vi "1.-Cubo RGB.vi"() -> ()   [LabVIEW 2020]
panel:
  out "new picture 6":picture
  out "RGB Cube Bottom":picture
  out "RGB Cube Right":picture
  out "RGB Cube Front":picture
  out "RGB Cube Left":picture
  out "RGB Cube Top":picture
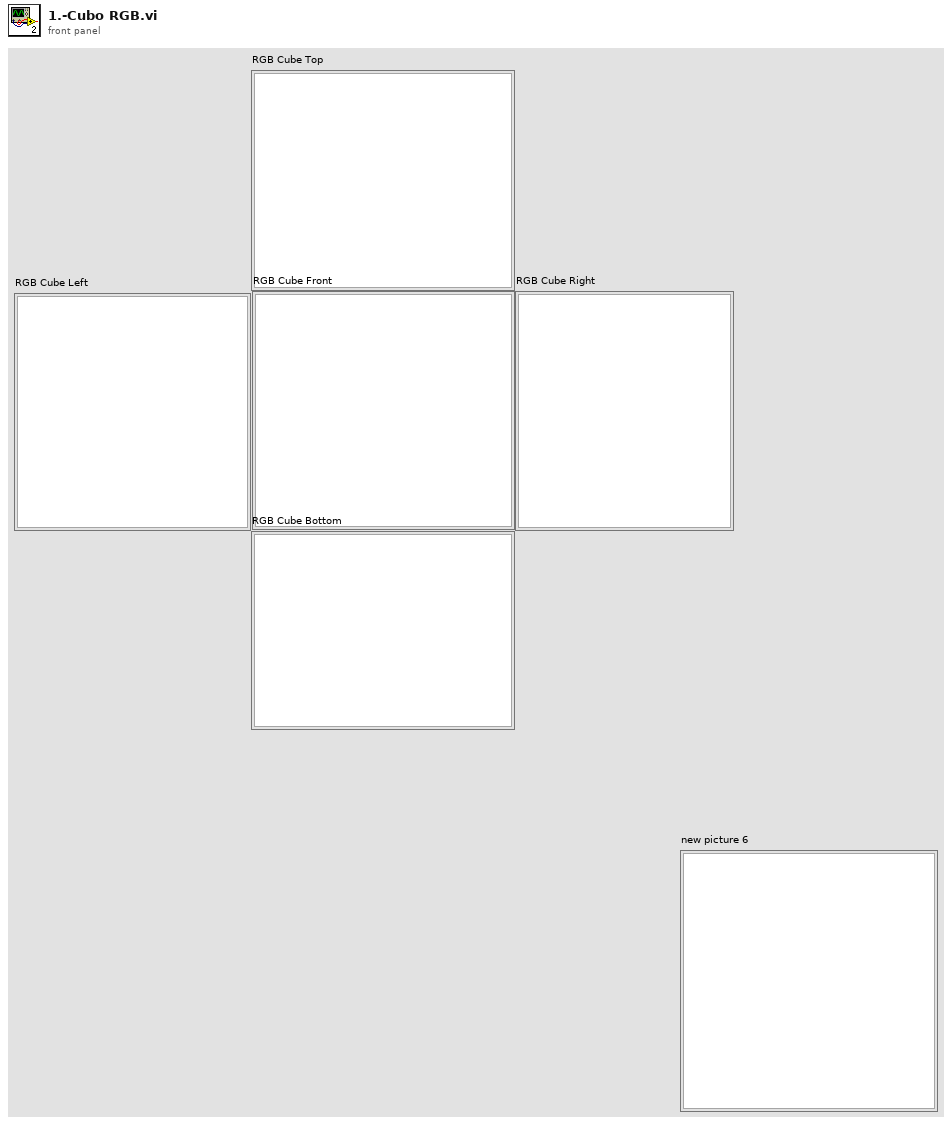
[diagram p1: front panel]
types:
  T1 = typedef "imagedata.ctl" = cluster{"image type":i32, "image depth":i32, "image":u8[], "mask":u8[], "colors":u32[], "Rectangle":cluster{"left":i16, "top":i16, "right":i16, "bottom":i16}}
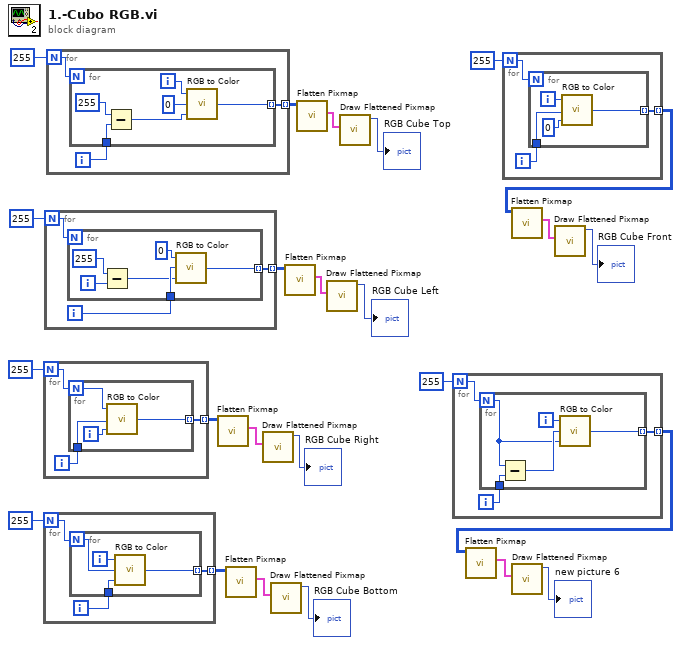
[diagram p0: block diagram]
diagram:
  n1 = for {
    N: 255 -> [w25]
    tunnel: [w26] -> w9 mode=indexing
    i -> [w27]
    n2 = for {
      N: w25 -> [w29]
      tunnel: w27 -> [w30]
      tunnel: [w31] -> w26 mode=indexing
      i -> [w28]
      n3 = call <vilib>:"RGB to Color.vi"("B"=w28, "G"=w30, "R"=w29) -> ("Color"=w31:u32)
    }
  }
  n4 = for {
    N: 255 -> [w32]
    tunnel: [w33] -> w5 mode=indexing
    i -> [w34]
    n5 = for {
      N: w32 -> [w36]
      tunnel: w34 -> [w35]
      tunnel: [w38] -> w33 mode=indexing
      i -> [w37]
      n6 = call <vilib>:"RGB to Color.vi"("B"=w35, "G"=w36, "R"=w37) -> ("Color"=w38:u32)
    }
  }
  n7 = for {
    N: 255 -> [w39]
    tunnel: [w40] -> w17 mode=indexing
    i -> [w41]
    n8 = for {
      N: w39 -> [_]
      tunnel: w41 -> [w44]
      tunnel: [w47] -> w40 mode=indexing
      i -> [w43]
      n9 = Subtract(x=255, y=w43) -> (x-y=w42:i32)
      n10 = call <vilib>:"RGB to Color.vi"("B"=w42, "G"=w44, "R"=0) -> ("Color"=w47:u32)
    }
  }
  n11 = for {
    N: 255 -> [w48]
    tunnel: [w49] -> w21 mode=indexing
    i -> [w50]
    n12 = for {
      N: w48 -> [_]
      tunnel: w50 -> [w53]
      tunnel: [w55] -> w49 mode=indexing
      i -> [w56]
      n13 = Subtract(x=255, y=w53) -> (x-y=w51:i32)
      n14 = call <vilib>:"RGB to Color.vi"("B"=w51, "G"=0, "R"=w56) -> ("Color"=w55:u32)
    }
  }
  n15 = call <vilib>:"Flatten Pixmap.vi"("24-bit pixmap"=w9) -> ("image data"=w11:T1)  [unwired: 10 in]
  n16 = call <vilib>:"Flatten Pixmap.vi"("24-bit pixmap"=w5) -> ("image data"=w7:T1)  [unwired: 10 in]
  n17 = call <vilib>:"Draw Flattened Pixmap.vi"("image data"=w11) -> ("new picture"=→"RGB Cube Right":picture)  [unwired: 8 in]
  n18 = call <vilib>:"Draw Flattened Pixmap.vi"("image data"=w7) -> ("new picture"=→"RGB Cube Bottom":picture)  [unwired: 8 in]
  n19 = call <vilib>:"Flatten Pixmap.vi"("24-bit pixmap"=w17) -> ("image data"=w19:T1)  [unwired: 10 in]
  n20 = call <vilib>:"Flatten Pixmap.vi"("24-bit pixmap"=w21) -> ("image data"=w23:T1)  [unwired: 10 in]
  n21 = call <vilib>:"Draw Flattened Pixmap.vi"("image data"=w19) -> ("new picture"=→"RGB Cube Left":picture)  [unwired: 8 in]
  n22 = call <vilib>:"Draw Flattened Pixmap.vi"("image data"=w23) -> ("new picture"=→"RGB Cube Top":picture)  [unwired: 8 in]
  n23 = for {
    N: 255 -> [w57]
    tunnel: [w58] -> w1 mode=indexing
    i -> [w59]
    n24 = for {
      N: w57 -> [w60]
      tunnel: w59 -> [w61]
      tunnel: [w64] -> w58 mode=indexing
      i -> [w63]
      n25 = Subtract(x=w60, y=w61) -> (x-y=w62:i32)
      n26 = call <vilib>:"RGB to Color.vi"("B"=w60, "G"=w62, "R"=w63) -> ("Color"=w64:u32)
    }
  }
  n27 = call <vilib>:"Flatten Pixmap.vi"("24-bit pixmap"=w1) -> ("image data"=w3:T1)  [unwired: 10 in]
  n28 = for {
    N: 255 -> [w65]
    tunnel: [w66] -> w13 mode=indexing
    i -> [w67]
    n29 = for {
      N: w65 -> [_]
      tunnel: w67 -> [w68]
      tunnel: [w71] -> w66 mode=indexing
      i -> [w70]
      n30 = call <vilib>:"RGB to Color.vi"("B"=0, "G"=w68, "R"=w70) -> ("Color"=w71:u32)
    }
  }
  n31 = call <vilib>:"Flatten Pixmap.vi"("24-bit pixmap"=w13) -> ("image data"=w15:T1)  [unwired: 10 in]
  n32 = call <vilib>:"Draw Flattened Pixmap.vi"("image data"=w3) -> ("new picture"=→"new picture 6":picture)  [unwired: 8 in]
  n33 = call <vilib>:"Draw Flattened Pixmap.vi"("image data"=w15) -> ("new picture"=→"RGB Cube Front":picture)  [unwired: 8 in]
